vi "Test SenseHat Basic.vi"() -> ()   [LabVIEW 2020]
uses:
  src/RPI.SenseHat/SenseHat/SenseHat.lvclass/SenseHat.ctl
  src/RPI.SenseHat/SenseHat/Get RPI.SenseHat.Joystick.vi
  src/RPI.SenseHat/SenseHat/Get RPI.SenseHat.Display.vi
  <vilib>/MakerHub/LINX/Public/Utilities/Open Local.vi
  src/RPI.SenseHat.Joystick/Classes/senseHatJoystick/RPI.SenseHat.Joystick.lvclass
  src/RPI.SenseHat.Display/Classes/SenseHat.Display/RPI.SenseHat.Display.lvclass
  <vilib>/MakerHub/LINX/LMH-LINX.lvlib
  src/RPI.SenseHat/SenseHat/SenseHat.lvclass
  src/RPI.SenseHat.Display/RPI.SenseHat.Display.lvlib
panel:
  out "Image":u32[][](array[colorbox])
  in  "Stop":bool
  out "Device Name":string
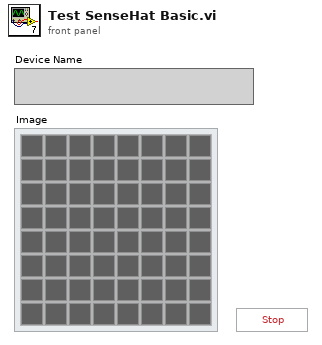
[diagram p1: front panel]
types:
  T1 = typedef "LMH-LINX.lvlib/LINX Ref.ctl" = cluster{"IO":T2, "Interface":T3, "LINX Device Config":T4}
  T2 = typedef "LMH-LINX.lvlib/Platform.ctl" = enum16{"Remote", "Local"}
  T3 = typedef "LMH-LINX.lvlib/Interface.ctl" = enum16{"Serial", "TCP"}
  T4 = typedef "LMH-LINX.lvlib/Device.lvlib/LINX Device Config.ctl" = cluster{"Interface":T3, "COM Port":refnum<visa-resource-name>, "TCP Configuration":T5, "Device Family":u8, "Device ID":u8, "Device Name":string, "TCP Ref":refnum<k5>, "Channels":T6}
  T5 = typedef "LMH-LINX.lvlib/Device.lvlib/TCP Config.ctl" = cluster{"IP Address":string, "Port":u16}
  T6 = typedef "LMH-LINX.lvlib/Channels.ctl" = cluster{"DI":u8[], "DO":u8[], "AI":u8[], "AO":u8[], "PWM":u8[], "QE":u8[], "UART":u8[], "I2C 2":u8[], "SPI":u8[], "CAN":u8[], "Servo":u8[], "AI Ref (V)":dbl, "AI Resolution (Bits)":u8, "AO Ref (V)":dbl, "AO Resolution (Bits)":u8}
  T7 = typedef "RPI.SenseHat.Joystick.lvlib/Joystick.ctl" = cluster{"Enter":bool, "Down":bool, "Up":bool, "Right":bool, "Left":bool}
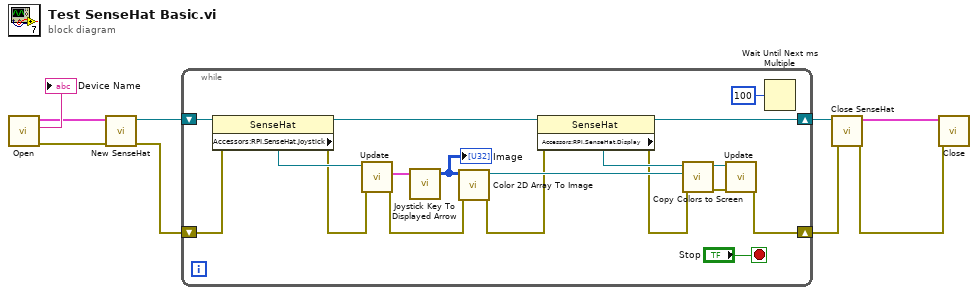
[diagram p0: block diagram]
diagram:
  n1 = call-poly <vilib>:"Open.vi"() -> ("Error Out"=w4:errorcluster, "Device Name"=→"Device Name":string, "LINX Resource"=w8:T1)  [unwired: 9 in]
  n2 = call "New SenseHat.vi"("error in (no error)"=w4, "LINX Resource"=w8) -> ("error out"=w3:errorcluster, "SenseHat out"=w6:refnum<class "SenseHat.lvclass">)  [unwired: 8 in]
  n3 = while {
    shift-right: [w23] -> w5
    shift-left: w6 -> [w26]
    shift-right: [w10] -> w2
    shift-left: w3 -> [w16]
    stop <- "Stop" stop-if-true
    n4 = property class="SenseHat"(reference=w26, error in=w16) -> (reference out=w25:refnum<class "SenseHat.lvclass">, error out=w15:errorcluster, "Accessors:RPI.SenseHat.Joystick"=w27:refnum<class "RPI.SenseHat.Joystick.lvclass">)
    n5 = call "Update.vi"("error in (no error)"=w15, "senseHatJoystick in"=w27) -> ("error out"=w14:errorcluster, "Joystick"=w19:T7)  [unwired: 7 in, 1 out]
    n6 = call "Joystick Key To Displayed Arrow.vi"("Joystick"=w19) -> ("Color[]"=w17:u32[][])  [unwired: 4 in]
    "Image" <- w17
    n7 = call "Color 2D Array To Image.vi"("error in (no error)"=w14, "Color[]"=w17) -> ("error out"=w12:errorcluster, "Image out"=w22:refnum<class "Image.lvclass">)  [unwired: 8 in]
    n8 = property class="SenseHat"(reference=w25, error in=w12) -> (reference out=w23:refnum<class "SenseHat.lvclass">, error out=w11:errorcluster, "Accessors:RPI.SenseHat.Display"=w24:refnum<class "RPI.SenseHat.Display.lvclass">)
    n9 = call "Copy Colors to Screen.vi"("error in (no error)"=w11, "Image"=w22, "senseHatDisplay in"=w24) -> ("error out"=w13:errorcluster, "senseHatDisplay out"=w18:refnum<class "RPI.SenseHat.Display.lvclass">)  [unwired: 7 in]
    n10 = call "Update.vi"("error in (no error)"=w13, "senseHatDisplay in"=w18) -> ("error out"=w10:errorcluster)  [unwired: 8 in, 1 out]
    n11 = Wait Until Next ms Multiple(millisecond multiple=u32 100) -> ()  [unwired: 1 out]
  }
  n12 = call "Close SenseHat.vi"("error in (no error)"=w2, "SenseHat in"=w5) -> ("error out"=w1:errorcluster, "LINX Resource"=w7:T1)  [unwired: 8 in]
  n13 = call <vilib>:"Close.vi"("Error In"=w1, "LINX Resource"=w7) -> ()  [unwired: 9 in, 1 out]
